vi "VITester_Provider_Shutdown.vi"(8 "error in (no error)":errorcluster, 10 "Is LV Exiting?":bool, 11 "Project Refnum":refnum<vi>) -> (0 "error out":errorcluster)   [LabVIEW 2009]
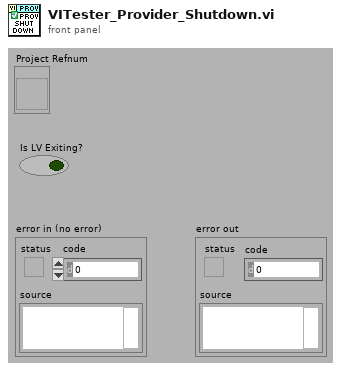
[diagram p1: front panel]
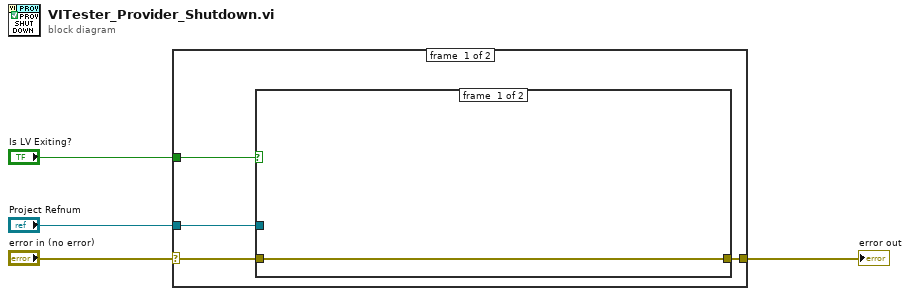
[diagram p0: block diagram]
diagram:
  n1 = case shown="No Error" "error in (no error)" {
    selector: "error in (no error)" -> [w7 w11]
    tunnel: [w6 w11] -> w3
    tunnel: "Is LV Exiting?" -> [w8 _]
    tunnel: "Project Refnum" -> [w5 _]
    frame #0 {
      n2 = case shown="True" w8 {
        tunnel: w7 -> [w9 w10]
        tunnel: [w9 w10] -> w6
        tunnel: w5 -> [_ _]
        frame #0 {
        }
        frame #1 {
        }
      }
    }
    frame #1 {
    }
  }
  "error out" <- w3
